vi "_db.vi"(7 "command":T2, 8 "error in (no error)":errorcluster, 10 "db in":T1, 11 "name":string) -> (0 "error out":errorcluster, 1 "created new?":bool, 3 "db out":T1, 4 "info":cluster{"db":T1, "Count":i32}, 6 "db list":string[](array[string]))   [LabVIEW 2014, in "TagDB(dev).lvlib"]
doc: "[Covers: REQ_TAGDB_NAMEDDB]"
uses:
  TagDB(dev).lvlib
  _DEF-DBOper.ctl
  tagDB_Def.ctl
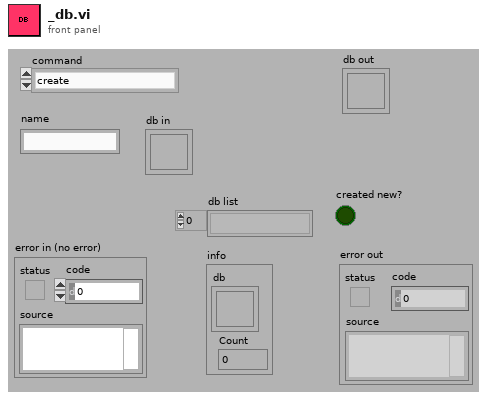
[diagram p1: front panel]
types:
  T1 = typedef "TagDB(dev).lvlib/tagDB_Def.ctl" = refnum<k1>
  T2 = typedef "TagDB(dev).lvlib/_DEF-DBOper.ctl" = enum16{"create", "destroy", "cleanUp", "list", "get info"}
  T3 = typedef "TagDB(dev).lvlib/_DEF-DATA.ctl" = cluster{"data hashmap":variant, "DataChangeFlag":i64, "ItemChangeFlag":i64, "name":string, "Tag Adding Lock?":bool}
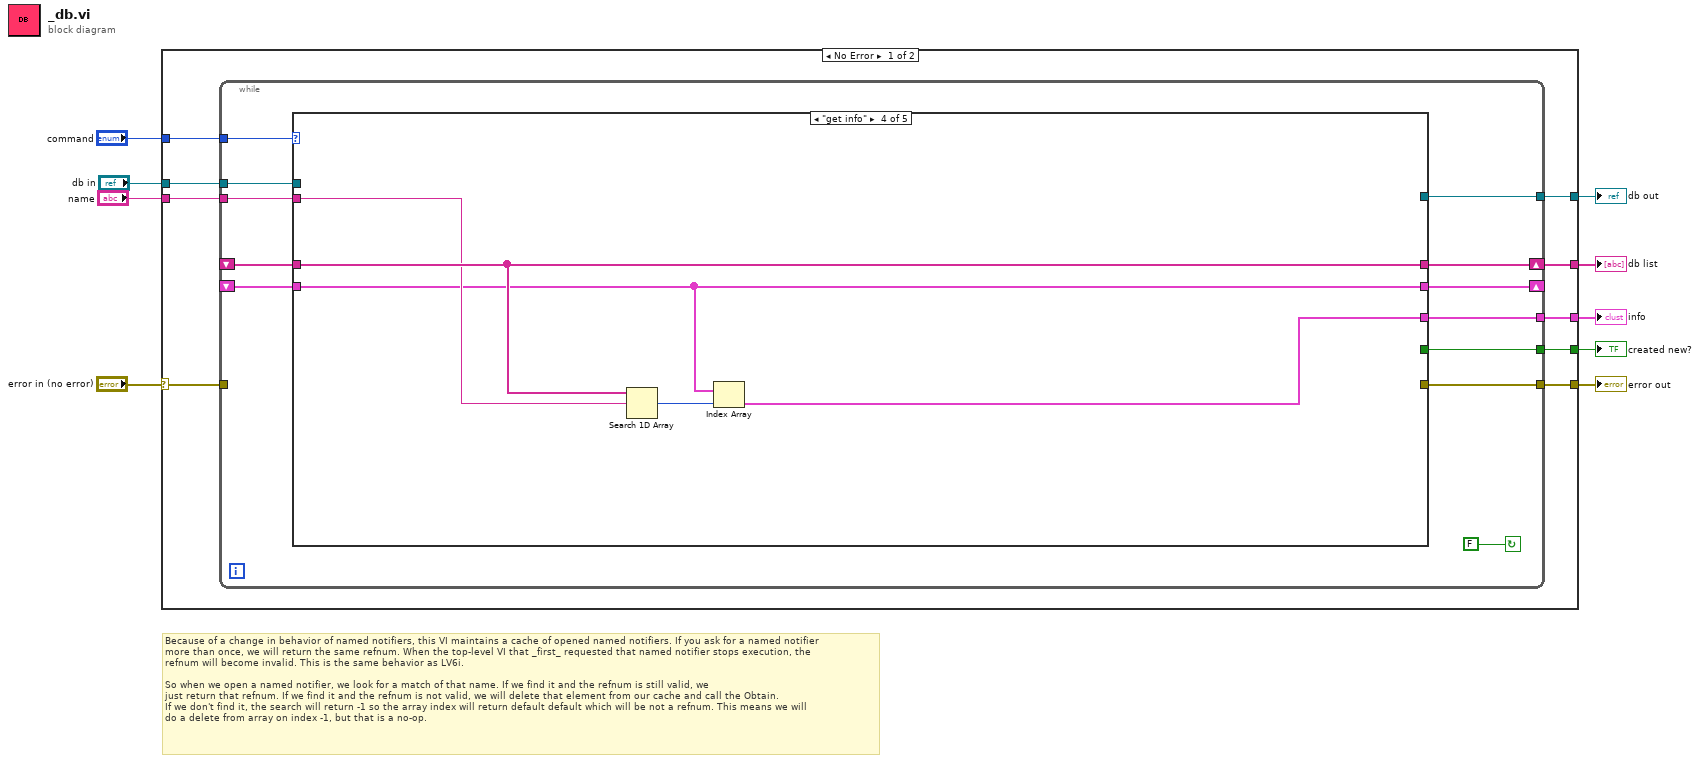
[diagram p0: block diagram]
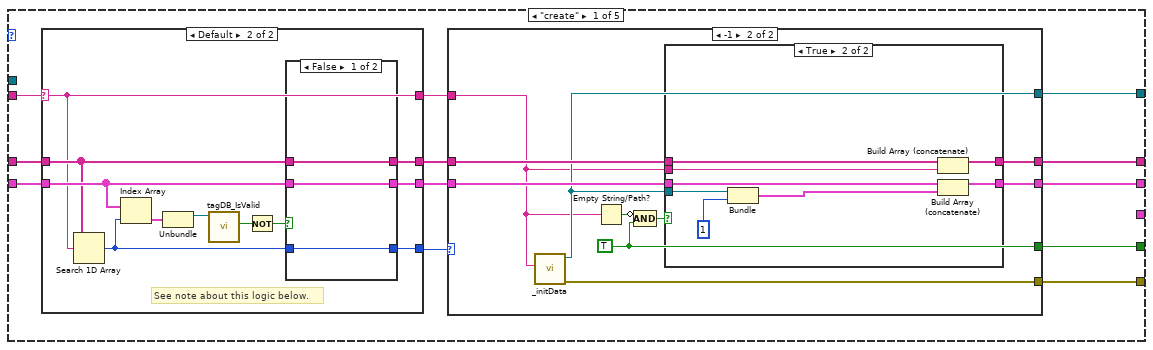
[diagram p2: hidden frame]
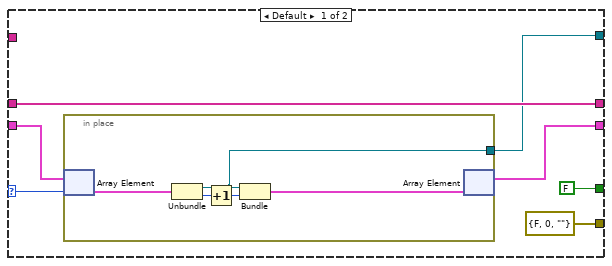
[diagram p3: hidden frame]
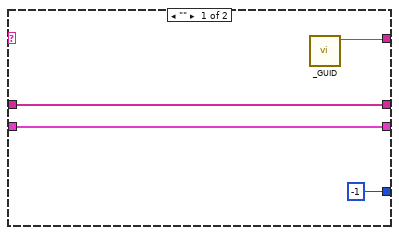
[diagram p5: hidden frame]
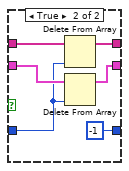
[diagram p6: hidden frame]
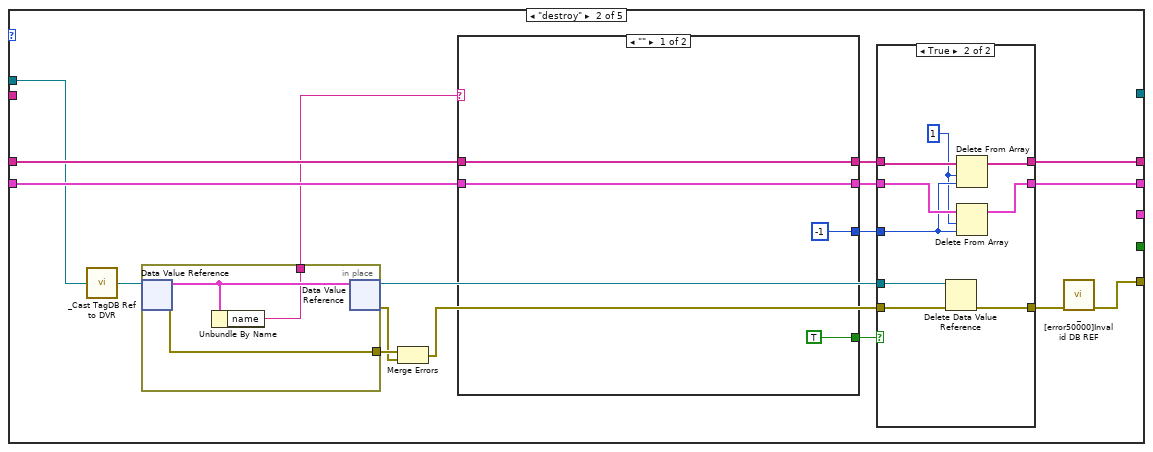
[diagram p7: hidden frame]
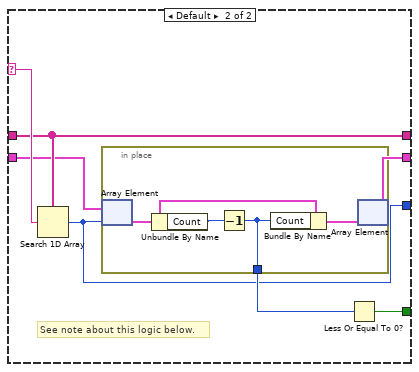
[diagram p9: hidden frame]
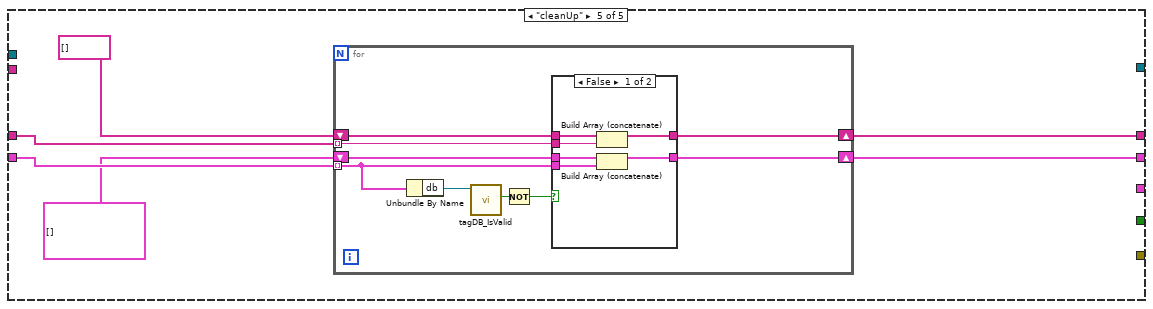
[diagram p11: hidden frame]
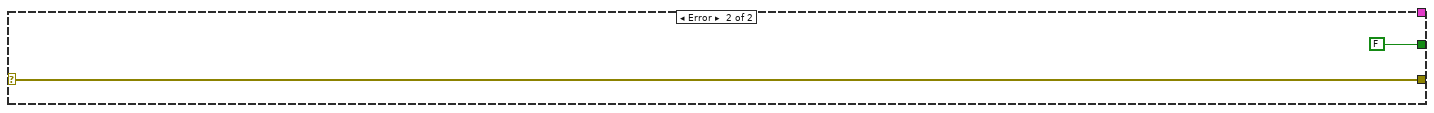
[diagram p13: hidden frame]
diagram:
  # "Because of a change in behavior of named notifiers, this VI maintains a cache of opened named notifiers. If you ask for a named notifier\nmore than once, we will return the same refnum. When the top-level VI that _first_ requested that named notifier stops execution, the\nrefnum will become invalid. This is the same behavior as LV6i.\n\nSo when we open a named notifier, we look for a match of that name. If we find it and the refnum is still valid, we\njust return that refnum. If we find it and the refnum is not valid, we will delete that element from our cache and call the Obtain.\nIf we don't find it, the search will return -1 so the array index will return default default which will be not a refnum. This means we will\ndo a delete from array on index -1, but that is a no-op."
  n1 = case shown="No Error" "error in (no error)" {
    selector: "error in (no error)" -> [w11 w177]
    tunnel: [w18 w177] -> w5
    tunnel: [w17 FALSE ("created new?")] -> w4
    tunnel: [w16 _] -> w9
    tunnel: "name" -> [w15 _]
    tunnel: "command" -> [w14 _]
    tunnel: "db in" -> [w13 _]
    tunnel: [w12 _] -> w2
    tunnel: [w10 _] -> w1
    frame No Error {
      n2 = while {
        shift-right: [w24] -> w12
        shift-left: _ -> [w30]
        shift-right: [w25] -> _
        shift-left: _ -> [w29]
        tunnel: [w28] -> w16
        tunnel: [w27] -> w18
        tunnel: [w26] -> w17
        tunnel: w15 -> [w22]
        tunnel: w14 -> [w19]
        tunnel: w13 -> [w21]
        tunnel: w11 -> [_]
        tunnel: [w20] -> w10
        stop <- FALSE continue-if-true
        n3 = case shown="\"get info\"" w19 {
          tunnel: w30 -> [w41 w115 w147 w152 w155]
          tunnel: w29 -> [w40 w114 w146 w150 w156]
          tunnel: [w39 _ _ _ _] -> w28
          tunnel: [w38 w105 _ _ _] -> w27
          tunnel: [w37 _ _ _ _] -> w26
          tunnel: [w34 w101 w146 w150 w157] -> w25
          tunnel: [w33 w103 w147 w152 w158] -> w24
          tunnel: w22 -> [w31 _ _ w151 _]
          tunnel: w21 -> [_ w110 _ _ _]
          tunnel: [_ _ _ w148 _] -> w20
          frame "create" {
            n4 = case shown="Default" w31 {
              selector: w31 -> [_ w83]
              tunnel: [w75 w83] -> w42
              tunnel: w41 -> [w78 w84]
              tunnel: w40 -> [w76 w89]
              tunnel: [w78 w88] -> w32
              tunnel: [w76 w87] -> w35
              tunnel: [-1 ("index") w86] -> w36
              frame "" {
                n5 = call "_GUID.vi"() -> ("uuid"=w75:string)  [unwired: 11 in]
              }
              frame Default {
                # "See note about this logic below."
                n6 = Search 1D Array(1D array=w84, element=w83) -> (index of element=w82:i32)  [unwired: 1 in]
                n7 = Index Array(array=w89, index=w82) -> (element=w81:cluster{"db":T1, "Count":i32})
                n8 = Unbundle(w81) -> ("db"=w79:T1)  [unwired: 1 out]
                n9 = call "tagDB_IsValid.vi"("DB Ref in"=w79) -> ("valid?"=w85:bool)  [unwired: 8 in, 2 out]
                n10 = Not(x=w85) -> (.not. x?=w80:bool)
                n11 = case shown="False" w80 {
                  tunnel: w82 -> [w90 w93]
                  tunnel: w89 -> [w92 w98]
                  tunnel: w84 -> [w91 w97]
                  tunnel: [w91 w96] -> w88
                  tunnel: [w92 w95] -> w87
                  tunnel: [w90 -1 ("index of element")] -> w86
                  frame False {
                  }
                  frame True {
                    n12 = Delete From Array(array=w97, index=w93) -> (array with subset deleted=w96:string[])  [unwired: 1 in, 1 out]
                    n13 = Delete From Array(array=w98, index=w93) -> (array with subset deleted=w95:cluster{"db":T1, "Count":i32}[])  [unwired: 1 in, 1 out]
                  }
                }
              }
            }
            n14 = case shown="-1" w36 {
              selector: w36 -> [w44 _]
              tunnel: w42 -> [_ w55]
              tunnel: [w46 w57] -> w39
              tunnel: [errorcluster {"status"=FALSE, "code"=0, "source"=""} ("error out") w64] -> w38
              tunnel: [FALSE ("created new?") w56] -> w37
              tunnel: w35 -> [w45 w60]
              tunnel: [w43 w61] -> w34
              tunnel: [w49 w62] -> w33
              tunnel: w32 -> [w49 w63]
              frame Default {
                n15 = in-place {
                  in-place-border: [w54] -> w46
                  n16 = in-place-array #1(w45, w44) -> (w51:cluster{"db":T1, "Count":i32})
                  n17 = Unbundle(w51) -> ("db"=w54:T1, "Count"=w53:i32)
                  n18 = Increment(x=w53) -> (x+1=w52:i32)
                  n19 = Bundle("db"=w54, w52) -> (w50:cluster{"db":T1, i32})  [unwired: 1 in]
                  n20 = in-place-array #1(w50) -> (w43:cluster{"db":T1, "Count":i32}[])  [unwired: 1 out]
                }
              }
              frame -1 {
                w56 = TRUE ("created new?")
                n21 = call "_initData.vi"("name"=w55) -> ("error out"=w64:errorcluster, "DB Ref(dup)"=w57:T1)  [unwired: 9 in]
                n22 = Empty String/Path?(string/path=w55) -> (empty?=w59:bool)
                n23 = Compound Arithmetic op=AND(invert w59, w56) -> (w58:bool)
                n24 = case shown="True" w58 {
                  tunnel: w63 -> [w66 w74]
                  tunnel: [w66 w72] -> w62
                  tunnel: [w65 w71] -> w61
                  tunnel: w60 -> [w65 w73]
                  tunnel: w57 -> [_ w68]
                  tunnel: w55 -> [_ w70]
                  frame False {
                  }
                  frame True {
                    n25 = Bundle("DB Ref(dup)"=w68, 1) -> (w69:cluster{"DB Ref(dup)":T1, i32})  [unwired: 1 in]
                    n26 = Build Array (concatenate)(w74, w70) -> (w72:string[])
                    n27 = Build Array (concatenate)(w73, w69) -> (w71:cluster{"DB Ref(dup)":T1, "Count":i32}[])
                  }
                }
              }
            }
          }
          frame "destroy" {
            n28 = call "_Cast TagDB Ref to DVR.vi"("TagDB"=w110) -> ("DVR"=w113:refnum<data-value>)  [unwired: 4 in]
            n29 = in-place {
              in-place-border: [w129] -> w112
              in-place-border: [w128] -> w109
              n30 = in-place-dvr #2(w113) -> (w130:T3, w129:errorcluster)
              n31 = Unbundle By Name(w130) -> ("name"=w128:string)
              n32 = in-place-dvr #2(w130) -> (w107:refnum<data-value>, w111:errorcluster)
            }
            n33 = Merge Errors(w112, w111) -> (w108:errorcluster)
            n34 = case shown="\"\"" w109 {
              selector: w109 -> [_ w141]
              tunnel: w115 -> [w134 w140]
              tunnel: w114 -> [w133 w136]
              tunnel: [w134 w140] -> w102
              tunnel: [w133 w137] -> w100
              tunnel: [TRUE w139] -> w104
              tunnel: [-1 ("index of element") w135] -> w99
              frame "" {
              }
              frame Default {
                # "See note about this logic below."
                n35 = Search 1D Array(1D array=w140, element=w141) -> (index of element=w135:i32)  [unwired: 1 in]
                n36 = in-place {
                  in-place-border: [w144] -> w138
                  n37 = in-place-array #3(w136, w135) -> (w142:cluster{"db":T1, "Count":i32})
                  n38 = Unbundle By Name(w142) -> ("Count"=w145:i32)
                  n39 = Decrement(x=w145) -> (x-1=w144:i32)
                  n40 = Bundle By Name(cluster=w142, "Count"=w144) -> (w143:cluster{"db":T1, "Count":i32})
                  n41 = in-place-array #3(w143) -> (w137:cluster{"db":T1, "Count":i32}[])  [unwired: 1 out]
                }
                n42 = Less Or Equal To 0?(x=w138) -> (x <= 0?=w139:bool)
              }
            }
            n43 = case shown="True" w104 {
              tunnel: w108 -> [w118 w127]
              tunnel: w107 -> [_ w126]
              tunnel: [w118 w125] -> w106
              tunnel: [w117 w123] -> w103
              tunnel: w102 -> [w117 w124]
              tunnel: [w116 w121] -> w101
              tunnel: w100 -> [w116 w122]
              tunnel: w99 -> [_ w120]
              frame False {
              }
              frame True {
                w119 = 1 ("length")
                n44 = Delete Data Value Reference(data value reference=w126, error in=w127) -> (error out=w125:errorcluster)  [unwired: 1 out]
                n45 = Delete From Array(array=w124, length=w119, index=w120) -> (array with subset deleted=w123:string[])  [unwired: 1 out]
                n46 = Delete From Array(array=w122, length=w119, index=w120) -> (array with subset deleted=w121:cluster{"db":T1, "Count":i32}[])  [unwired: 1 out]
              }
            }
            n47 = call "_[error50000]Invalid DB REF.vi"("error in (no error)"=w106) -> ("error out"=w105:errorcluster)  [unwired: 10 in]
          }
          frame "list" {
          }
          frame "get info" {
            n48 = Search 1D Array(1D array=w152, element=w151) -> (index of element=w149:i32)  [unwired: 1 in]
            n49 = Index Array(array=w150, index=w149) -> (element=w148:cluster{"db":T1, "Count":i32})
          }
          frame "cleanUp" {
            n50 = for {
              shift-right: [w166] -> w158
              shift-left: string[] [] -> [w167]
              tunnel: w156 -> [w161] mode=indexing
              shift-right: [w165] -> w157
              shift-left: cluster{"db":T1, "Count":i32}[] [] -> [w163]
              tunnel: w155 -> [w164] mode=indexing
              n51 = Unbundle By Name(w161) -> ("db"=w159:T1)
              n52 = call "tagDB_IsValid.vi"("DB Ref in"=w159) -> ("valid?"=w162:bool)  [unwired: 8 in, 2 out]
              n53 = Not(x=w162) -> (.not. x?=w160:bool)
              n54 = case shown="False" w160 {
                tunnel: w167 -> [w173 w175]
                tunnel: w161 -> [w169 _]
                tunnel: [w172 w175] -> w166
                tunnel: [w170 w174] -> w165
                tunnel: w164 -> [w171 _]
                tunnel: w163 -> [w168 w174]
                frame False {
                  n55 = Build Array (concatenate)(w173, w171) -> (w172:string[])
                  n56 = Build Array (concatenate)(w168, w169) -> (w170:cluster{"db":T1, "Count":i32}[])
                }
                frame True {
                }
              }
            }
          }
        }
      }
    }
    frame Error {
    }
  }
  "created new?" <- w4
  "error out" <- w5
  "db out" <- w9
  "db list" <- w2
  "info" <- w1
